vi "Create Signal Sessions (SubVI).vi"(8 "error in":errorcluster, 10 "Select":bool, 11 "macrotick offset":u32) -> (0 "error out":errorcluster, 3 "Sessions":T1, 5 "timing source out":string)   [LabVIEW 2010]
uses:
  Sessions.ctl
  <vilib>/xnet/xnet.llb/XNET Create Session (Signal Input Single-point).vi
  <vilib>/xnet/xnet.llb/XNET Create Session (Signal Output Single-point).vi
  <vilib>/xnet/xnet.llb/XNET Create Timing Source (FlexRay Cycle).vi
  Program Files (x86)/National Instruments/LabVIEW 2010/resource/objmgr/xnet.rc
panel:
  # "Send SigA and recieve SigC"
  # "Send SigC and recieve SigA"
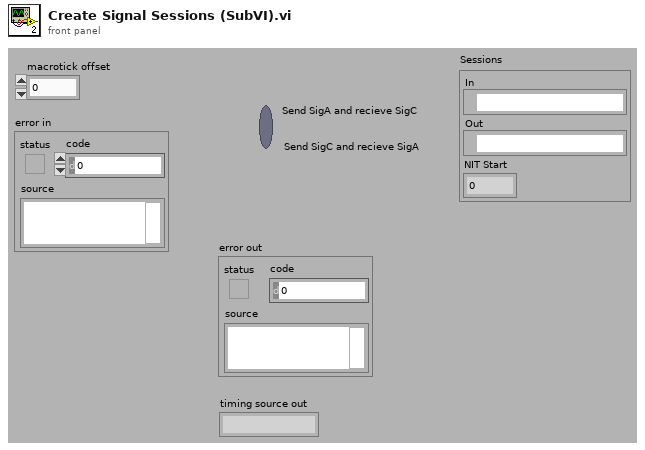
[diagram p1: front panel]
types:
  T1 = typedef "Sessions.ctl" = cluster{"In":refnum<k21>, "Out":refnum<k21>, "NIT Start":u32}
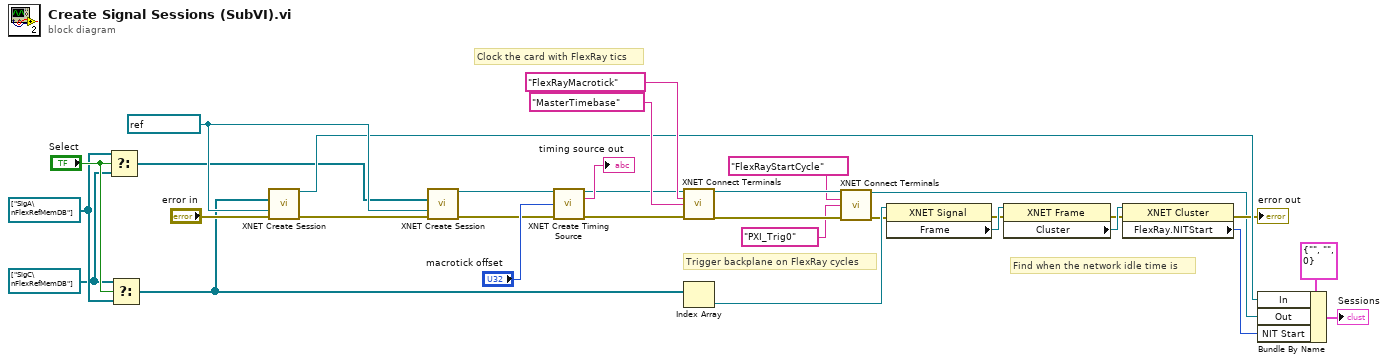
[diagram p0: block diagram]
diagram:
  w17 = refnum<k21>[] ["SigC\nFlexRefMemDB"] ("signal list")
  w18 = refnum<k21>[] ["SigA\nFlexRefMemDB"] ("signal list")
  w23 = refnum<k21> "FlexRay1" ("interface")
  # "Find when the network idle time is"
  # "Clock the card with FlexRay tics"
  # "Trigger backplane on FlexRay cycles"
  n1 = Select(t=w18, s="Select", f=w17) -> (s? t:f=w16:refnum<k21>[])
  n2 = Select(t=w17, s="Select", f=w18) -> (s? t:f=w10:refnum<k21>[])
  n3 = call-poly <vilib>:"XNET Create Session.vi"("signal list"=w10, "interface"=w23, "error in (no error)"="error in") -> ("session out"=w21:refnum<k21>, "error out"=w24:errorcluster)  [unwired: 11 in]
  n4 = call-poly <vilib>:"XNET Create Session.vi"("signal list"=w16, "interface"=w23, "error in (no error)"=w24) -> ("session out"=w26:refnum<k21>, "error out"=w25:errorcluster)  [unwired: 11 in]
  n5 = call-poly <vilib>:"XNET Create Timing Source.vi"("session in"=w26, "macrotick offset"="macrotick offset", "error in (no error)"=w25) -> ("session out"=w29:refnum<k21>, "timing source out"=→"timing source out":string, "error out"=w28:errorcluster)  [unwired: 10 in]
  n6 = call <vilib>:"XNET Connect Terminals.vi"("session in"=w29, "source terminal"=tag "FlexRayMacrotick" ("XNET Terminal"), "destination terminal"=tag "MasterTimebase" ("XNET Terminal"), "error in (no error)"=w28) -> ("session out"=w5:refnum<k21>, "error out"=w6:errorcluster)  [unwired: 10 in]
  n7 = Index Array(array=w10) -> (element=w9:refnum<k21>)  [unwired: 1 in]
  n8 = call <vilib>:"XNET Connect Terminals.vi"("session in"=w5, "source terminal"=tag "FlexRayStartCycle", "destination terminal"=tag "PXI_Trig0" ("source terminal"), "error in (no error)"=w6) -> ("session out"=w1:refnum<k21>, "error out"=w4:errorcluster)  [unwired: 10 in]
  n9 = property class="XNET Signal"(reference=w9, error in=w4) -> (error out=w13:errorcluster, "Frame"=w15:refnum<k21>)  [unwired: 1 out]
  n10 = property class="XNET Frame"(reference=w15, error in=w13) -> (error out=w12:errorcluster, "Cluster"=w14:refnum<k21>)  [unwired: 1 out]
  n11 = property class="XNET Cluster"(reference=w14, error in=w12) -> (error out=→"error out":errorcluster, "FlexRay.NITStart"=w7:u32)  [unwired: 1 out]
  n12 = Bundle By Name(cluster=T1 {"In"="", "Out"="", "NIT Start"=0} ("Sessions"), "In"=w21, "Out"=w1, "NIT Start"=w7) -> (→"Sessions":T1)
